vi "Best_Match.vi"(2 "Input String":string, 3 "String Options":string[](array[string])) -> (0 "Good Match":bool, 1 "index of element":i32)   [LabVIEW 2011]
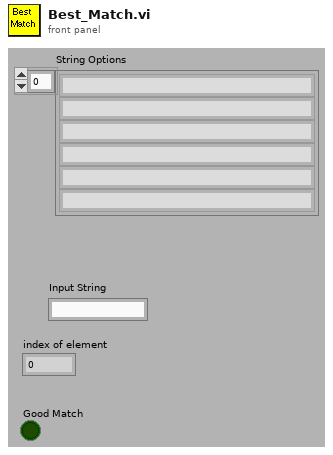
[diagram p1: front panel]
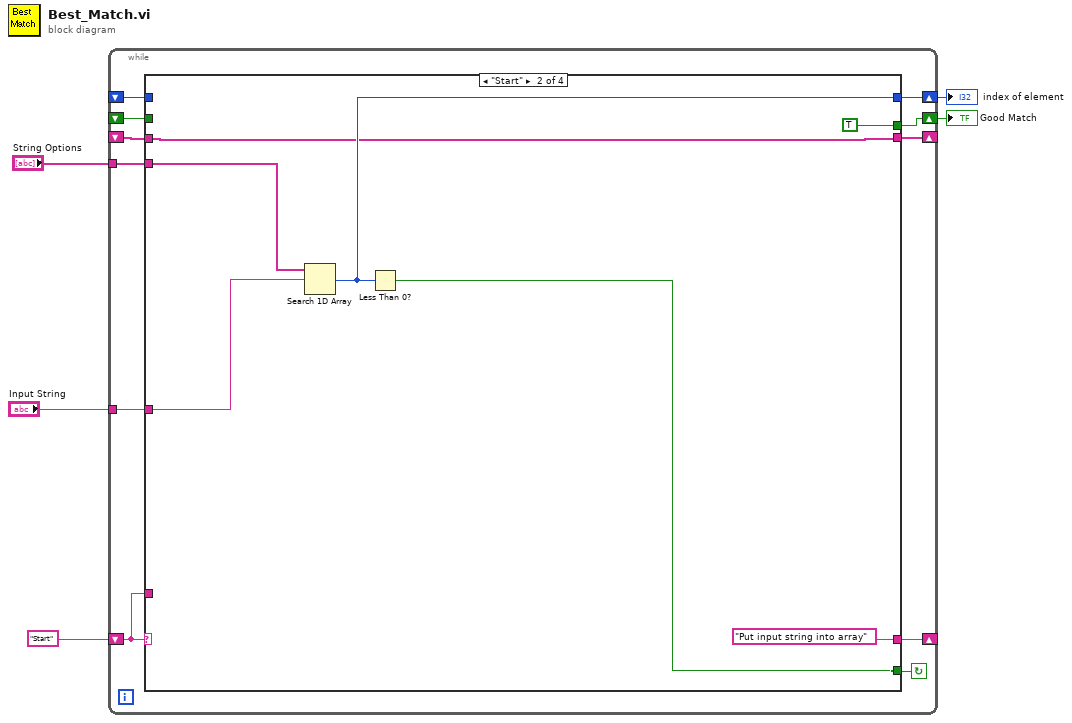
[diagram p0: block diagram]
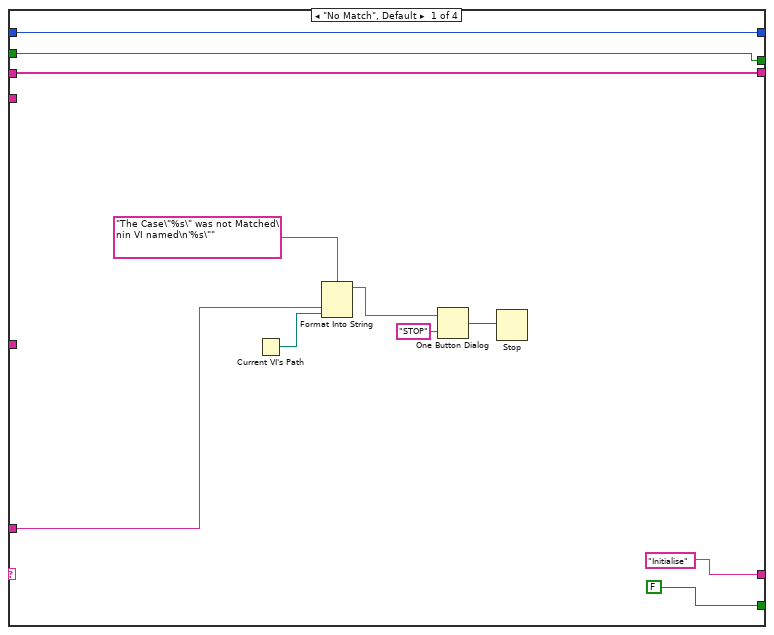
[diagram p2: hidden frame]
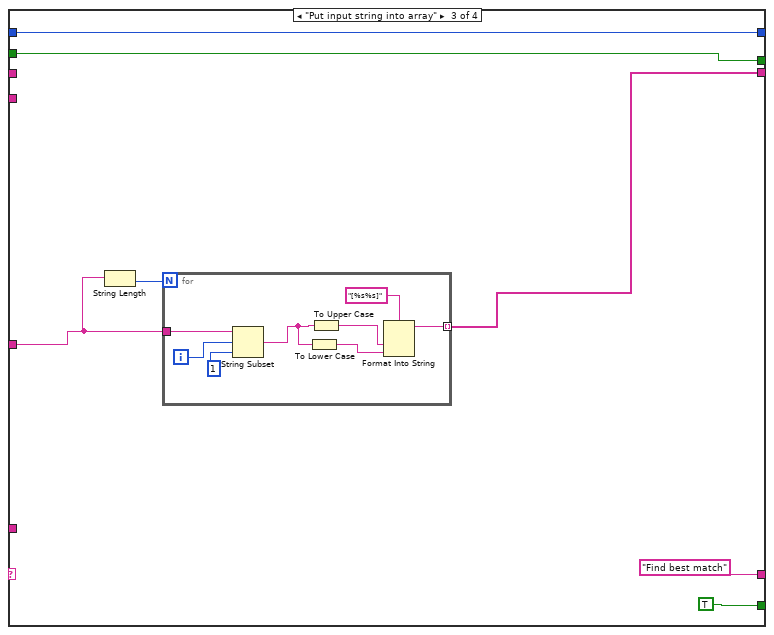
[diagram p3: hidden frame]
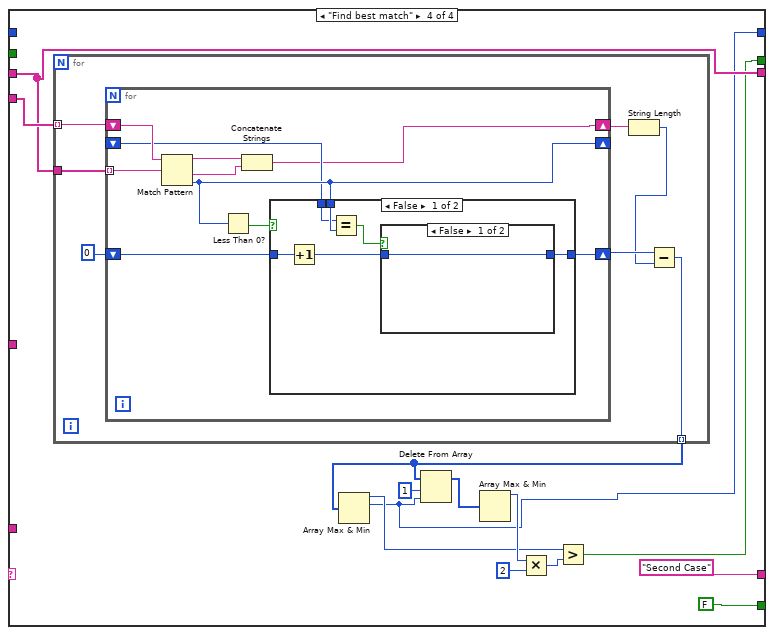
[diagram p4: hidden frame]
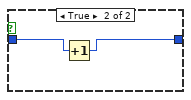
[diagram p5: hidden frame]
diagram:
  n1 = while {
    shift-left: "Start" -> [w14]
    shift-right: [w15] -> _
    tunnel: "String Options" -> [w13]
    tunnel: "Input String" -> [w12]
    shift-right: [w11] -> w2
    shift-left: _ -> [w9]
    shift-right: [w10] -> w1
    shift-left: _ -> [w8]
    shift-right: [w7] -> _
    shift-left: _ -> [w6]
    stop <- w16 continue-if-true
    n2 = case shown="\"Start\"" w14 {
      tunnel: [FALSE w31 TRUE FALSE] -> w16
      tunnel: ["Initialise" "Put input string into array" "Find best match" "Second Case"] -> w15
      tunnel: w14 -> [w22 _ _ _]
      tunnel: w13 -> [_ w33 _ w60]
      tunnel: w12 -> [_ w32 w39 _]
      tunnel: [w19 w30 w36 w51] -> w11
      tunnel: [w18 TRUE w35 w50] -> w10
      tunnel: w9 -> [w19 _ w36 _]
      tunnel: w8 -> [w18 _ w35 _]
      tunnel: [w17 w29 w37 w59] -> w7
      tunnel: w6 -> [w17 w29 _ w59]
      frame "No Match", Default {
        n3 = Current VI's Path() -> (path=w21:path)
        n4 = Format Into String(format string="The Case\"%s\" was not Matched\nin VI named\n'%s\"" ("Format String"), w22, w21) -> (resulting string=w25:string)  [unwired: 2 in, 1 out]
        n5 = One Button Dialog(message=w25, button name ("OK")="STOP") -> (true=w23:bool)
        n6 = Stop(stop? (T)=w23) -> ()
      }
      frame "Start" {
        n7 = Search 1D Array(1D array=w33, element=w32) -> (index of element=w30:i32)  [unwired: 1 out]
        n8 = Less Than 0?(x=w30) -> (x < 0?=w31:bool)
      }
      frame "Put input string into array" {
        n9 = String Length(string=w39) -> (length=w38:i32)
        n10 = for {
          N: w38 -> [_]
          tunnel: w39 -> [w48]
          tunnel: [w42] -> w37 mode=indexing
          i -> [w43]
          n11 = String Subset(string=w48, offset (0)=w43, length (rest)=1 ("length (rest)")) -> (substring=w47:string)
          n12 = To Lower Case(string=w47) -> (all lower case string=w45:string)
          n13 = To Upper Case(1:w47) -> (0:w46:string)
          n14 = Format Into String(format string="[%s%s]", w46, w45) -> (resulting string=w42:string)  [unwired: 2 in, 1 out]
        }
      }
      frame "Find best match" {
        n15 = for {
          tunnel: w59 -> [w69]
          tunnel: w60 -> [w68] mode=indexing
          tunnel: [w63] -> w58 mode=indexing
          n16 = for {
            tunnel: w69 -> [w79] mode=indexing
            shift-right: [w70] -> w66
            shift-left: w68 -> [w78]
            shift-right: [w72] -> _
            shift-left: _ -> [w71]
            shift-right: [w74] -> w65
            shift-left: 0 -> [w73]
            n17 = Match Pattern(string=w78, regular expression=w79) -> (before substring=w77:string, after substring=w76:string, offset past match=w72:i32)  [unwired: 2 out]
            n18 = Less Than 0?(x=w72) -> (x < 0?=w75:bool)
            n19 = Concatenate Strings(w77, w76) -> (w70:string)
            n20 = case shown="False" w75 {
              tunnel: [w80 w89] -> w74
              tunnel: w73 -> [w85 w89]
              tunnel: w72 -> [w84 _]
              tunnel: w71 -> [w83 _]
              frame False {
                n21 = Increment(x=w85) -> (x+1=w81:i32)
                n22 = Equal?(x=w83, y=w84) -> (x = y?=w82:bool)
                n23 = case shown="False" w82 {
                  tunnel: w81 -> [w86 w88]
                  tunnel: [w86 w87] -> w80
                  frame False {
                  }
                  frame True {
                    n24 = Increment(x=w88) -> (x+1=w87:i32)
                  }
                }
              }
              frame True {
              }
            }
          }
          n25 = String Length(string=w66) -> (length=w64:i32)
          n26 = Subtract(x=w65, y=w64) -> (x-y=w63:i32)
        }
        n27 = Array Max & Min(array=w58) -> (max value=w52:i32, max index (indices)=w51:i32)  [unwired: 2 out]
        n28 = Delete From Array(array=w58, length=1, index=w51) -> (array with subset deleted=w56:i32[])  [unwired: 1 out]
        n29 = Array Max & Min(array=w56) -> (max value=w55:i32)  [unwired: 3 out]
        n30 = Multiply(x=w55, y=2) -> (x*y=w53:i32)
        n31 = Greater?(x=w52, y=w53) -> (0:w50:bool)
      }
    }
  }
  "index of element" <- w2
  "Good Match" <- w1
